vi "test drone.vi"() -> ()   [LabVIEW 2018]
uses:
  <vilib>/vision/Image Controls.llb/IMAQ Image.ctl
  <vilib>/Utility/error.llb/Error Cluster From Error Code.vi
  <vilib>/myRIO/Common/Instrument Driver Framework/myRIO v1.0/DIO/vis/myRIO v1.0 Write DIO.vi
  <vilib>/myRIO/Common/Instrument Driver Framework/myRIO v1.0/PWM/vis/myRIO v1.0 Write PWM.vi
  <vilib>/vision/driver/NI_Vision_Acquisition_Software.lvlib
  <vilib>/vision/NI_Vision_Development_Module.lvlib
  <vilib>/myRIO/Instrument Drivers/Onboard IO/PWM/PWM.lvlib
  <vilib>/myRIO/Instrument Drivers/Onboard IO/DIO/DIO.lvlib
panel:
  in  "Gimbal search":bool
  in  "Stop":bool
  out "Image 5":T1(plugin-control)
  out "Y":dbl[](array[numeric])
  out "X":dbl[](array[numeric])
  out "Antal isbjerg":i32
  out "logfile name":path
  in  "logfile base name":string="logfile"
  in  "Color Plane (Color Plane Extraction 1)":i32(ring)=1 items=["Red", "Green", "Blue", "Hue", "Saturation", "Luminance", "Value", "Intensity"]
  in  "Range (Threshold 1)":cluster{"Lower value":sgl, "Upper value":sgl}={"Lower value"=230.0, "Upper value"=255.0}
  in  "Structuring Element (Basic Morphology 1)":i32[][](array[numeric])=[[0, 1, 0], [1, 1, 1], [0, 1, 0]]
  in  "Number of Erosion (Advanced Morphology 1)":i32=12
  in  "Grounded?":bool
  in  "Pos. ROLL Boring":dbl
  in  "Pos. YAW Boring":dbl format="%#_13g"
  in  "Pos. ROLL No Search":dbl
  in  "Pos. YAW No Search":dbl format="%#_13g"
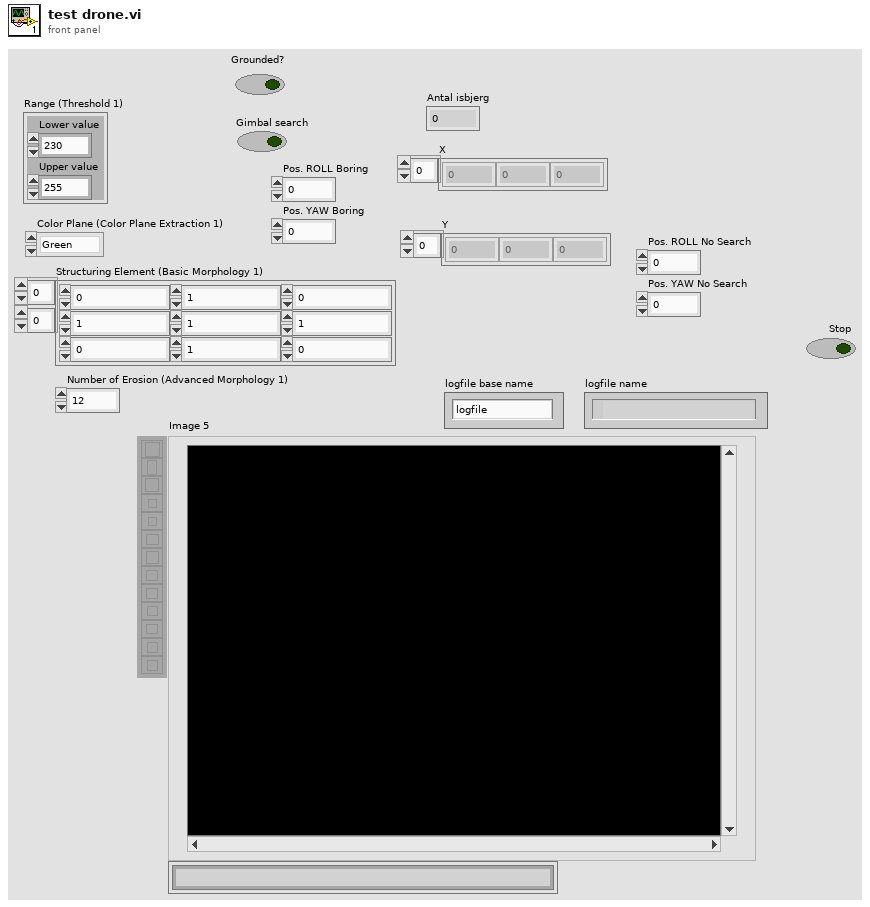
[diagram p1: front panel]
types:
  T1 = typedef "IMAQ Image.ctl" = refnum<image>
  T2 = typedef "DIO.lvlib/DIO Reference.ctl" = cluster{"myRIO Reference":T3, "DIO Channels List":T7}
  T3 = typedef "myRIO Generic Hardware Reference.ctl" = cluster{"myRIO Model":T4, "myRIO Hardware Reference":T5}
  T4 = typedef "Hardware Version Enum.ctl" = enum16{"Unknown", "myRIO-1900", "myRIO-1950", "roboRIO", "NI ELVIS RIO CM", "ELVIS III"}
  T5 = typedef "myRIO v1.0 Reference.ctl" = cluster{"Generic FPGA Reference":T6, "Allow multiple opens":bool}
  T6 = typedef "Generic FPGA Reference.ctl" = refnum<k20>
  T7 = typedef "DIO Channels List.ctl" = T8[]
  T8 = typedef "DIO Channels Enum.ctl" = enum16{"Not Connected", "C/DIO0", "C/DIO1", "C/DIO2", "C/DIO3", "C/DIO4", "C/DIO5", "C/DIO6", "C/DIO7", "A/DIO0", "A/DIO1", "A/DIO2", "A/DIO3", "A/DIO4", "A/DIO5", "A/DIO6", "A/DIO7", "A/DIO8", "A/DIO9", "A/DIO10", "A/DIO11", "A/DIO12", "A/DIO13", "A/DIO14", "A/DIO15", "A/DIO16", "A/DIO17", "A/DIO18", "A/DIO19", "B/DIO0", "B/DIO1", "B/DIO2", "B/DIO3", "B/DIO4", "B/DIO5", "B/DIO6", "B/DIO7", "B/DIO8", "B/DIO9", "B/DIO10", "B/DIO11", "B/DIO12", "B/DIO13", "B/DIO14", "B/DIO15", "B/DIO16", "B/DIO17", "B/DIO18", "B/DIO19", "LED0", "LED1", "LED2", "LED3", "Button0", "DIO/DIO0", "DIO/DIO1", "DIO/DIO2", "DIO/DIO3", "DIO/DIO4", "DIO/DIO5", "DIO/DIO6", "DIO/DIO7", "DIO/DIO8", "DIO/DIO9", "SPI/CS0", "SPI/CS1", "SPI/CS2", "SPI/CS3", "LED RADIO (Green)", "LED RADIO (Red)", "LED COMM (Green)", "LED COMM (Red)", "LED MODE (Green)", "LED MODE (Red)"}
  T9 = typedef "PWM.lvlib/PWM Reference.ctl" = cluster{"myRIO Reference":T3, "PWM Channels Enum":T10, "PWM Configuration":T11}
  T10 = typedef "PWM Channels Enum.ctl" = enum16{"Not Connected", "C/PWM0", "C/PWM1", "A/PWM0", "A/PWM1", "A/PWM2", "A/PWM3", "A/PWM4", "A/PWM5", "A/PWM6", "A/PWM7", "A/PWM8", "A/PWM9", "A/PWM10", "A/PWM11", "A/PWM12", "A/PWM13", "A/PWM14", "A/PWM15", "A/PWM16", "A/PWM17", "A/PWM18", "A/PWM19", "B/PWM0", "B/PWM1", "B/PWM2", "B/PWM3", "B/PWM4", "B/PWM5", "B/PWM6", "B/PWM7", "B/PWM8", "B/PWM9", "B/PWM10", "B/PWM11", "B/PWM12", "B/PWM13", "B/PWM14", "B/PWM15", "B/PWM16", "B/PWM17", "B/PWM18", "B/PWM19", "PWM/PWM0", "PWM/PWM1", "PWM/PWM2", "PWM/PWM3", "PWM/PWM4", "PWM/PWM5", "PWM/PWM6", "PWM/PWM7", "PWM/PWM8", "PWM/PWM9"}
  T11 = typedef "PWM.lvlib/PWM Configuration.ctl" = cluster{"Frequency":dbl, "Duty Cycle":dbl}
  T12 = typedef "Accelerometer.lvlib/Accelerometer Reference.ctl" = cluster{"myRIO Reference":T3, "Accelerometer Channels List":T13, "LSB Weight":dbl}
  T13 = typedef "Accelerometer Channels List.ctl" = T14[]
  T14 = typedef "Accelerometer Channels Enum.ctl" = enum16{"Not Connected", "X-Axis", "Y-Axis", "Z-Axis"}
  T15 = typedef "AI.lvlib/AI Reference.ctl" = cluster{"myRIO Reference":T3, "AI Channels List":T16, "AI Scaling Constants List":T18}
  T16 = typedef "AI Channels List.ctl" = T17[]
  T17 = typedef "AI Channels Enum.ctl" = enum16{"Not Connected", "AudioIn/Left", "AudioIn/Right", "C/AI0", "C/AI1", "A/AI0", "A/AI1", "A/AI2", "A/AI3", "A/AI4", "A/AI5", "A/AI6", "A/AI7", "B/AI0", "B/AI1", "B/AI2", "B/AI3", "B/AI4", "B/AI5", "B/AI6", "B/AI7", "AI/AI0", "AI/AI1", "AI/AI2", "AI/AI3", "A/AI0 (DIFF)", "A/AI1 (DIFF)", "A/AI2 (DIFF)", "A/AI3 (DIFF)", "B/AI0 (DIFF)", "B/AI1 (DIFF)", "B/AI2 (DIFF)", "B/AI3 (DIFF)"}
  T18 = typedef "Analog Scaling Constants List.ctl" = T19[]
  T19 = typedef "Analog Scaling Constants.ctl" = cluster{"LSB Weight (Volts)":dbl, "Offset (Volts)":dbl, "Signed?":bool}
  T20 = typedef "SPI.lvlib/SPI Reference.ctl" = cluster{"myRIO Reference":T3, "SPI Channels Enum":T21, "SPI Configuration":T22}
  T21 = typedef "SPI Channels Enum.ctl" = enum16{"Not Connected", "A/SPI", "B/SPI", "SPI/SPI"}
  T22 = typedef "SPI.lvlib/SPI Configuration.ctl" = cluster{"Frequency [Hz]":dbl, "Clock Phase":T23, "Clock Polarity":T24, "Data Direction":T25, "Frame Length":T26}
  T23 = typedef "SPI Clock Phase.ctl" = enum8{"Leading", "Trailing"}
  T24 = typedef "SPI Clock Polarity.ctl" = enum8{"Low", "High"}
  T25 = typedef "SPI Data Direction.ctl" = enum8{"Most significant bit first", "Least significant bit first"}
  T26 = typedef "SPI Frame Length.ctl" = u8
  T27 = cluster{"B/DIO0 - Stepper Direction":T2, "B/DIO1 - Stepper1 Enable":T2, "B/DIO2 - Stepper2 Enable":T2, "B/DIO3 - Stepper3 Enable":T2, "B/DIO4 - Endstop Stepper1 Top":T2, "B/DIO11 - Endstop Stepper1 Bund":T2, "B/DIO12 - Endstop Stepper2 Top":T2, "B/DIO13 - Endstop Stepper2 Bund":T2, "B/DIO14 - Endstop Stepper3 Top":T2, "B/DIO15 - Endstop Stepper3 Bund":T2, "A/DIO0 - Cooler":T2, "A/DIO1 - Beacon drop (dio1)":T2, "A/DIO2 - Beacon drop (dio0)":T2, "A/DIO3 - QuickRelease (dio1)":T2, "A/DIO4 - QuickRelease (dio0)":T2, "A/DIO11 - LiDAR SPI CS":T2, "B/PWM0 - Stepper":T9, "B/PWM1 - Drill":T9, "A/PWM0 - Servo_Roll":T9, "A/PWM1 - Servo_Yaw":T9, "Acc. X-axis":T12, "Acc. Y-axis":T12, "B/AI0 - Drone Grounded F3":T15, "B/AI1 - Drone Drill Gear F4":T15, "B/AI2 - Beacon Drop F5":T15, "B/AI3 - Drone Drill Boost F6":T15, "A/AI0 - Drone Stepper F8":T15, "A/AI1 - Beacon Wiper":T15, "A/AI2 - QuickRelease Wiper":T15, "A/AI3 - Drill Current":T15, "A/SPI - LiDAR":T20, "B/UART - XBee":refnum<visa-resource-name>, "A/UART - A3 GPS":refnum<visa-resource-name>, "RIO Flashing LEDs":T2}
  T28 = enum32{"AutoM", "Close", "Dilate", "Erode", "Gradient", "Gradient out", "Gradient in", "Hit miss", "Open", "PClose", "POpen", "Thick", "Thin"}
  T29 = typedef "Image Type" = u32
  T30 = typedef "IMAQdx.ctl" = refnum<k21>
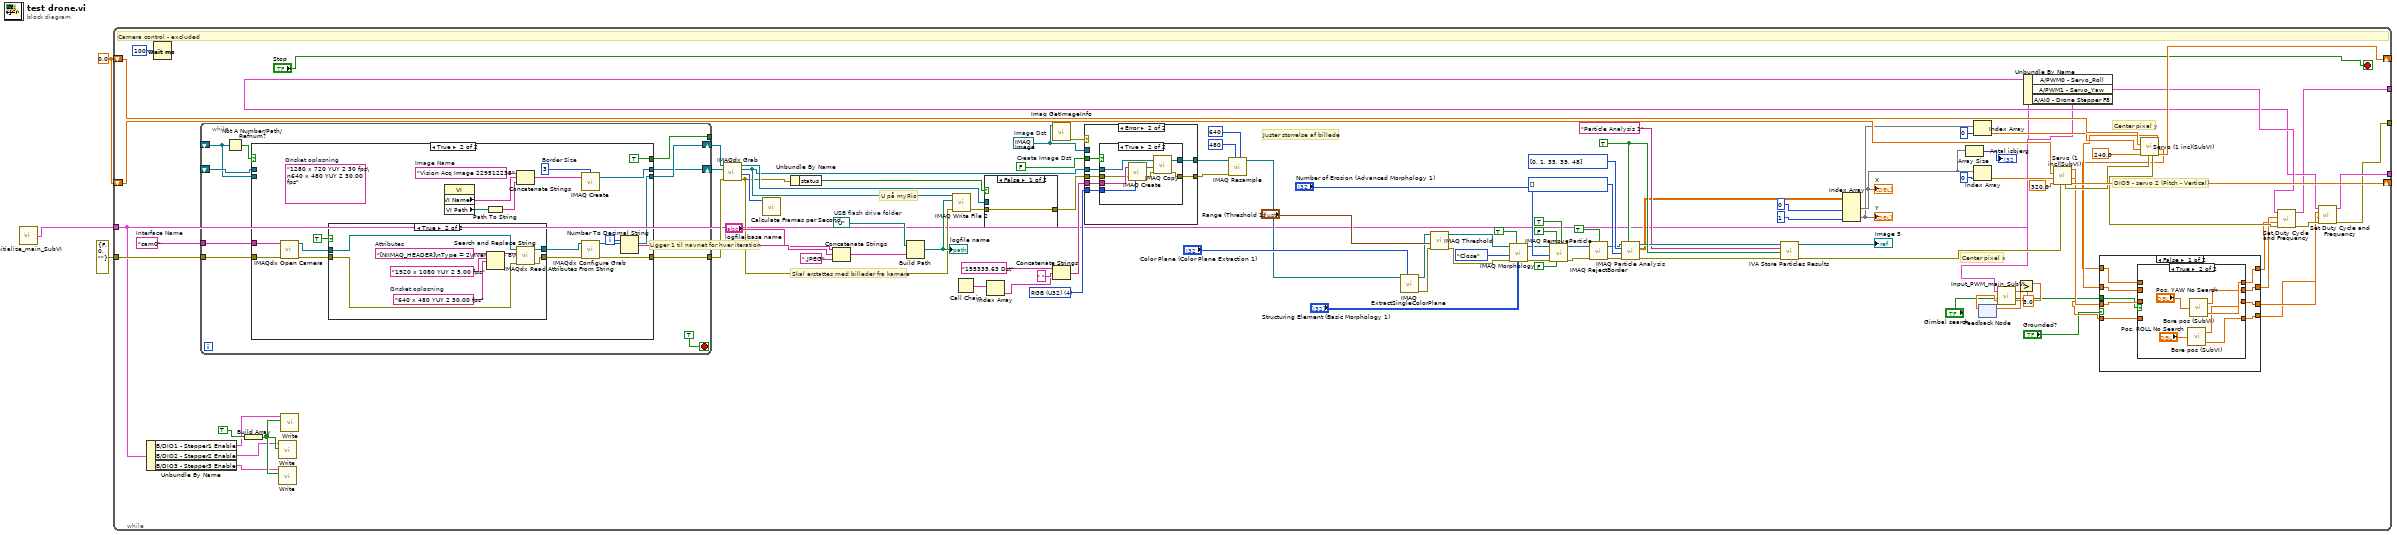
[diagram p0: block diagram]
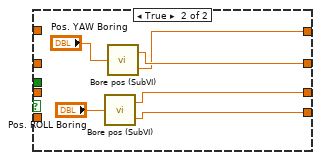
[diagram p3: hidden frame]
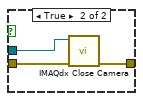
[diagram p4: hidden frame]
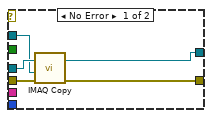
[diagram p7: hidden frame]
diagram:
  w1 = 0.0 ("Position 2")
  n1 = call "Initialize_main_SubVI.vi"() -> ("output cluster"=w3:T27)
  n2 = while {
    shift-right: [w78] -> _
    shift-left: w1 -> [w81]
    shift-right: [w93] -> _
    shift-left: w1 -> [w94]
    tunnel: errorcluster {"status"=FALSE, "code"=0, "source"=""} ("error out") -> [w95]
    tunnel: w3 -> [w10]
    tunnel: [w30] -> _
    tunnel: [w34] -> _
    tunnel: [w33] -> _
    i -> [w68]
    stop <- "Stop" stop-if-true
    w46 = i32[] [] items=["Center of Mass X", "Center of Mass Y", "First Pixel X", "First Pixel Y", "Bounding Rect Left", "Bounding Rect Top", "Bounding Rect Right", "Bounding Rect Bottom", "Max Feret Diameter Start X", "Max Feret Diameter Start Y", "Max Feret Diameter End X", "Max Feret Diameter End Y", "Max Horiz. Segment Length Left", "Max Horiz. Segment Length Right", "Max Horiz. Segment Length Row", "-", "Bounding Rect Width", "Bounding Rect Height", "Bounding Rect Diagonal", "Perimeter", "Convex Hull Perimeter", "Holes' Perimeter", "Max Feret Diameter", "Equivalent Ellipse Major Axis", "Equivalent Ellipse Minor Axis", "Equivalent Ellipse Minor Axis (Feret)", "Equivalent Rect Long Side", "Equivalent Rect Short Side", "Equivalent Rect Diagonal", "Equivalent Rect Short Side (Feret)", "Average Horiz. Segment Length", "Average Vert. Segment Length", "Hydraulic Radius", "Waddel Disk Diameter", "-", "Area", "Holes' Area", "Particle & Holes' Area", "Convex Hull Area", "Image Area", "-", "Number of Holes", "Number of Horiz. Segments", "Number of Vert. Segments", "-", "Orientation", "Max Feret Diameter Orientation", "-", "% Area/Image Area", "% Area/(Particle & Holes' Area)", "Ratio of Equivalent Ellipse Axes", "Ratio of Equivalent Rect Sides", "-", "Elongation Factor", "Compactness Factor", "Heywood Circularity Factor", "Type Factor", "-", "Sum X", "Sum Y", "Sum XX", "Sum XY", "Sum YY", "Sum XXX", "Sum XXY", "Sum XYY", "Sum YYY", "-", "Moment of Inertia XX", "Moment of Inertia XY", "Moment of Inertia YY", "Moment of Inertia XXX", "Moment of Inertia XXY", "Moment of Inertia XYY", "Moment of Inertia YYY", "Norm. Moment of Inertia XX", "Norm. Moment of Inertia XY", "Norm. Moment of Inertia YY", "Norm. Moment of Inertia XXX", "Norm. Moment of Inertia XXY", "Norm. Moment of Inertia XYY", "Norm. Moment of Inertia YYY", "Hu Moment 1", "Hu Moment 2", "Hu Moment 3", "Hu Moment 4", "Hu Moment 5", "Hu Moment 6", "Hu Moment 7"] ("Real-World Measurements")
    w47 = i32[] [0, 1, 35, 39, 48] items=["Center of Mass X", "Center of Mass Y", "First Pixel X", "First Pixel Y", "Bounding Rect Left", "Bounding Rect Top", "Bounding Rect Right", "Bounding Rect Bottom", "Max Feret Diameter Start X", "Max Feret Diameter Start Y", "Max Feret Diameter End X", "Max Feret Diameter End Y", "Max Horiz. Segment Length Left", "Max Horiz. Segment Length Right", "Max Horiz. Segment Length Row", "-", "Bounding Rect Width", "Bounding Rect Height", "Bounding Rect Diagonal", "Perimeter", "Convex Hull Perimeter", "Holes' Perimeter", "Max Feret Diameter", "Equivalent Ellipse Major Axis", "Equivalent Ellipse Minor Axis", "Equivalent Ellipse Minor Axis (Feret)", "Equivalent Rect Long Side", "Equivalent Rect Short Side", "Equivalent Rect Diagonal", "Equivalent Rect Short Side (Feret)", "Average Horiz. Segment Length", "Average Vert. Segment Length", "Hydraulic Radius", "Waddel Disk Diameter", "-", "Area", "Holes' Area", "Particle & Holes' Area", "Convex Hull Area", "Image Area", "-", "Number of Holes", "Number of Horiz. Segments", "Number of Vert. Segments", "-", "Orientation", "Max Feret Diameter Orientation", "-", "% Area/Image Area", "% Area/(Particle & Holes' Area)", "Ratio of Equivalent Ellipse Axes", "Ratio of Equivalent Rect Sides", "-", "Elongation Factor", "Compactness Factor", "Heywood Circularity Factor", "Type Factor", "-", "Sum X", "Sum Y", "Sum XX", "Sum XY", "Sum YY", "Sum XXX", "Sum XXY", "Sum XYY", "Sum YYY", "-", "Moment of Inertia XX", "Moment of Inertia XY", "Moment of Inertia YY", "Moment of Inertia XXX", "Moment of Inertia XXY", "Moment of Inertia XYY", "Moment of Inertia YYY", "Norm. Moment of Inertia XX", "Norm. Moment of Inertia XY", "Norm. Moment of Inertia YY", "Norm. Moment of Inertia XXX", "Norm. Moment of Inertia XXY", "Norm. Moment of Inertia XYY", "Norm. Moment of Inertia YYY", "Hu Moment 1", "Hu Moment 2", "Hu Moment 3", "Hu Moment 4", "Hu Moment 5", "Hu Moment 6", "Hu Moment 7"] ("Pixel Measurements")
    w44 = TRUE ("Connectivity 4/8 (8)")
    w67 = path "U:/"  # USB flash drive folder
    w101 = "cam0"  # Interface Name
    w111 = T1 refnum  # Image Dst
    w103 = T29 4 items=["Grayscale (U8)", "Grayscale (I16)", "Grayscale (SGL)", "Complex (CSG)", "RGB (U32)", "HSL (U32)", "RGB (U64)", "Grayscale (U16)"] ("Image Dst Type")
    w109 = FALSE  # Create Image Dst
    # "Juster størrelse af billede"
    # "U på myRio"
    # "Ligger 1 til navnet for hver iteration"
    # "Skal erstattes med billeder fra kamera"
    # "Center pixel y"
    # "Center pixel x"
    # "DIO9 - servo 2 (Pitch - Vertical)"
    # "Camera control - excluded"
    n3 = Unbundle By Name(w10) -> ("B/DIO1 - Stepper1 Enable"=w7:T2, "B/DIO2 - Stepper2 Enable"=w6:T2, "B/DIO3 - Stepper3 Enable"=w5:T2)
    n4 = Wait (ms)(milliseconds to wait=u32 100) -> ()  [unwired: 1 out]
    n5 = while "While Loop_template0" {
      shift-right: [w150] -> w96
      shift-left: _ -> [w143]
      tunnel: [w149] -> w102
      tunnel: w95 -> [w148]
      shift-right: [w146] -> w97
      shift-left: _ -> [w145]
      tunnel: w101 -> [w144]
      tunnel: [w141] -> _
      stop <- TRUE ("_template0") stop-if-true
      n6 = Not A Number/Path/Refnum?(number/path/refnum=w143) -> (NaN/Path/Refnum?=w142:bool)
      n7 = case "Case Structure_template0" shown="True" w142 {
        tunnel: [w153 w169] -> w150
        tunnel: w143 -> [w153 _]
        tunnel: [w152 w168] -> w149
        tunnel: w148 -> [w152 w170]
        tunnel: [w151 w167] -> w146
        tunnel: w145 -> [w151 _]
        tunnel: w144 -> [_ w158]
        tunnel: [_ TRUE] -> w141
        frame False {
        }
        frame True {
          (unwired) "1280 x 720 YUY 2 30 fps\n640 x 480 YUY 2 30.00 fps"  # Ønsket opløsning
          w155 = 3  # Border Size
          w162 = "Vision Acq Image 229512235"  # Image Name
          n8 = call <vilib>:"IMAQdx Open Camera.vi"("error in"=w170, "Session In"=w158) -> ("error out"=w160:errorcluster, "Session Out"=w161:T30)  [unwired: 1 in, 7 out]
          n9 = case shown="True" TRUE ("Init Attributes") {
            tunnel: w161 -> [w172 w180]
            tunnel: w160 -> [w171 w179]
            tunnel: [w172 w178] -> w154
            tunnel: [w171 w177] -> w159
            frame False {
            }
            frame True {
              w173 = "640 x 480 YUY 2 30.00 fps"  # Ønsket opløsning
              w176 = "[NIIMAQ_HEADER]\nType = 2\nVersion = 8\n\n[CAMERA_DATA]\nAcquisitionAttributes::Bayer::Algorithm = \"Bilinear\"\nAcquisitionAttributes::Bayer::GainB = \"1\"\nAcquisitionAttributes::Bayer::GainG = \"1\"\nAcquisitionAttributes::Bayer::GainR = \"1\"\nAcquisitionAttributes::Bayer::Pattern = \"Use hardware value\"\nAcquisitionAttributes::BitsPerPixel = \"Use hardware value\"\nAcquisitionAttributes::HardwareMaximumQueuedBufferCount = \"1000\"\nAcquisitionAttributes::HardwareRequeueBufferListThreshold = \"50\"\nAcquisitionAttributes::IgnoreFirstFrame = \"false\"\nAcquisitionAttributes::ImageDecoderCopyMode = \"Auto\"\nAcquisitionAttributes::OutputImageType = \"Auto\"\nAcquisitionAttributes::OverwriteMode = \"Get Newest\"\nAcquisitionAttributes::PixelSignedness = \"Use hardware value\"\nAcquisitionAttributes::ReceiveTimestampMode = \"None\"\nAcquisitionAttributes::ShiftPixelBits = \"false\"\nAcquisitionAttributes::SwapPixelBytes = \"false\"\nAcquisitionAttributes::Timeout = \"5000\"\nAcquisitionAttributes::VideoMode = \"1920 x 1080 YUY 2 5.00 fps\"\nCameraAttributes::BacklightCompensation::Mode = \"Manual\"\nCameraAttributes::BacklightCompensation::Value = \"0\"\nCameraAttributes::Brightness::Mode = \"Manual\"\nCameraAttributes::Brightness::Value = \"168\"\nCameraAttributes::Contrast::Mode = \"Manual\"\nCameraAttributes::Contrast::Value = \"5\"\nCameraAttributes::Exposure::Mode = \"AutoAperaturePriority\"\nCameraAttributes::Focus::Mode = \"Auto\"\nCameraAttributes::Pan::Mode = \"Manual\"\nCameraAttributes::Pan::Value = \"0\"\nCameraAttributes::PowerLineFrequency::Mode = \"60Hz\"\nCameraAttributes::Saturation::Mode = \"Manual\"\nCameraAttributes::Saturation::Value = \"103\"\nCameraAttributes::Sharpness::Mode = \"Manual\"\nCameraAttributes::Sharpness::Value = \"25\"\nCameraAttributes::Tilt::Mode = \"Manual\"\nCameraAttributes::Tilt::Value = \"0\"\nCameraAttributes::WhiteBalance::Mode = \"Auto\"\nCameraAttributes::Zoom::Mode = \"Manual\"\nCameraAttributes::Zoom::Value = \"0\"\n"  # Attributes
              n10 = Search and Replace String(input string=w176, search string="1920 x 1080 YUY 2 5.00 fps", replace string=w173) -> (result string=w174:string)  [unwired: 5 in, 3 out]
              n11 = call <vilib>:"IMAQdx Read Attributes From String.vi"("error in"=w179, "Attributes String In"=w174, "Session In"=w180) -> ("error out"=w177:errorcluster, "Session Out"=w178:T30)  [unwired: 7 out]
            }
          }
          n12 = property class="VI"() -> ("VI Name"=w165:string, "VI Path"=w166:path)  [unwired: 2 in, 2 out]
          n13 = Path To String(path=w166) -> (string=w164:string)
          n14 = Concatenate Strings(w162, w165, w164) -> (w163:string)
          n15 = call "IMAQ Create"("Border Size"=w155, "Image Name"=w163) -> ("New Image"=w167:T1)  [unwired: 2 in, 2 out]
          n16 = call <vilib>:"IMAQdx Configure Grab.vi"("error in"=w159, "Session In"=w154) -> ("error out"=w168:errorcluster, "Session Out"=w169:T30)  [unwired: 8 out]
        }
      }
    }
    n17 = Build Array(TRUE) -> (w8:bool[])
    n18 = call <vilib>:"Write.vi"("Values"=w8, "DIO Ref In"=w6) -> ()  [unwired: 7 in, 2 out]
    n19 = call <vilib>:"Write.vi"("Values"=w8, "DIO Ref In"=w5) -> ()  [unwired: 7 in, 2 out]
    n20 = call <vilib>:"Write.vi"("Values"=w8, "DIO Ref In"=w7) -> ()  [unwired: 7 in, 2 out]
    n21 = Number To Decimal String(number=w68) -> (decimal integer string=w73:string)  [unwired: 1 in]
    n22 = call <vilib>:"IMAQdx Grab.vi"("error in"=w102, "Image In"=w97, "Session In"=w96) -> ("error out"=w70:errorcluster, "Buffer Number Out"=w100:u32, "Image Out"=w71:T1, "Session Out"=w99:T30)  [unwired: 1 in, 4 out]
    n23 = call <vilib>:"Calculate Frames per Second.vi"("Buffer Number"=w100) -> ()  [unwired: 2 in, 9 out]
    n24 = Unbundle By Name(w70) -> ("status"=w90:bool)
    n25 = Concatenate Strings "Concatenate Strings"("logfile base name", w73, ".JPEG" ("string")) -> (w75:string)
    n26 = Build Path(base path=w67, name or relative path=w75) -> (appended path=w76:path)
    "logfile name" <- w76
    n27 = call-poly "IMAQ Write File 2"("error in (no error)"=w70, "File Path"=w76, "Image"=w71) -> ("error out"=w69:errorcluster)  [unwired: 7 in, 1 out]
    n28 = Call Chain() -> (call chain=w108:string[])
    n29 = case "Case Structure_template1" shown="False" w90 {
      tunnel: [w137 w139] -> w98
      tunnel: w69 -> [w137 w140]
      tunnel: w99 -> [_ w138]
      frame False {
      }
      frame True {
        n30 = call <vilib>:"IMAQdx Close Camera.vi"("error in"=w140, "Session In"=w138) -> ("error out"=w139:errorcluster)  [unwired: 9 out]
      }
    }
    n31 = Index Array(array=w108) -> (element=w106:string)  [unwired: 1 in]
    n32 = call "Imaq GetImageInfo"("Image"=w111) -> ("error out"=w110:errorcluster)  [unwired: 1 in, 9 out]
    n33 = Concatenate Strings("155335,63 Dst" ("Image Dst Name"), " ", w106) -> (w104:string)
    n34 = case shown="Error" w110 {
      tunnel: [w185 w189] -> w38
      tunnel: [w184 w188] -> w37
      tunnel: w71 -> [w183 w190]
      tunnel: w98 -> [w182 w186]
      tunnel: w111 -> [w181 _]
      tunnel: w104 -> [_ w192]
      tunnel: w103 -> [_ w191]
      tunnel: w109 -> [_ w187]
      frame No Error {
        n35 = call "IMAQ Copy"("error in (no error)"=w182, "Image Dst"=w181, "Image Src"=w183) -> ("error out"=w184:errorcluster, "Image Dst Out"=w185:T1)  [unwired: 3 out]
      }
      frame Error {
        n36 = case shown="True" w187 {
          tunnel: w192 -> [_ w202]
          tunnel: w191 -> [_ w201]
          tunnel: w190 -> [w194 w199]
          tunnel: [w194 w198] -> w189
          tunnel: [w193 w197] -> w188
          tunnel: w186 -> [w193 w195]
          frame False {
          }
          frame True {
            n37 = call "IMAQ Create"("Image Name"=w202, "Image Type"=w201, "error in (no error)"=w195) -> ("New Image"=w200:T1, "error out"=w196:errorcluster)  [unwired: 1 in, 1 out]
            n38 = call "IMAQ Copy"("error in (no error)"=w196, "Image Dst"=w200, "Image Src"=w199) -> ("error out"=w197:errorcluster, "Image Dst Out"=w198:T1)  [unwired: 3 out]
          }
        }
      }
    }
    n39 = call "IMAQ Resample"("X Resolution"=u16 640 ("Width"), "Y Resolution"=u16 480 ("Height"), "error in (no error)"=w37, "Image Src"=w38) -> ("Image Dst Out"=w14:T1)  [unwired: 6 in, 1 out]
    n40 = call "IMAQ ExtractSingleColorPlane"("Color Plane"="Color Plane (Color Plane Extraction 1)", "Image Src"=w14) -> ("error out"=w65:errorcluster, "Image Dst Out"=w63:T1)  [unwired: 2 in, 6 out]
    n41 = call "IMAQ Threshold"("error in (no error)"=w65, "Range"="Range (Threshold 1)", "Image Src"=w63) -> ("error out"=w62:errorcluster, "Image Dst Out"=w58:T1)  [unwired: 3 in, 4 out]
    n42 = call "IMAQ Morphology"("Structuring Element"="Structuring Element (Basic Morphology 1)", "Square/Hexa (Square)"=TRUE, "error in (no error)"=w62, "Operation"=T28."Close", "Image Src"=w58) -> ("error out"=w57:errorcluster, "Image Dst Out"=w52:T1)  [unwired: 2 in, 3 out]
    n43 = call "IMAQ RemoveParticle"("Connectivity 4/8 (8)"=TRUE, "Low Pass/High Pass (Low)"=FALSE, "Square/Hexa (Square)"=FALSE, "error in (no error)"=w57, "Number of Erosion"="Number of Erosion (Advanced Morphology 1)", "Image Src"=w52) -> ("error out"=w51:errorcluster, "Image Dst Out"=w49:T1)  [unwired: 1 in, 3 out]
    n44 = call "IMAQ RejectBorder"("error in (no error)"=w51, "Image Src"=w49, "Connectivity 4/8 (8)"=TRUE) -> ("error out"=w48:errorcluster, "Image Dst Out"=w45:T1)  [unwired: 1 in, 2 out]
    n45 = call "IMAQ Particle Analysis"("Connectivity 4/8 (8)"=w44, "error in (no error)"=w48, "Real-World Measurements"=w46, "Pixel Measurements"=w47, "Image"=w45) -> ("error out"=w41:errorcluster, "Particle Measurements (Pixels)"=w39:dbl[][], "Image Out (duplicate)"=w43:T1)  [unwired: 4 out]
    n46 = call <vilib>:"IVA Store Particles Results.vi"("error in (no error)"=w41, "Connectivity 4/8 (8)"=w44, "Step Name"="Particle Analysis 1", "Image in"=w43) -> ("error out"=w40:errorcluster, "Image dup"=→"Image 5":T1)  [unwired: 6 out]
    n47 = Index Array(array=w39, index (col) #1=0 ("index (col)"), index (col) #2=1 ("index (col)")) -> (element #1=w85:dbl[], element #2=w82:dbl[])  [unwired: 2 in]
    "Y" <- w82
    "X" <- w85
    n48 = Array Size(array=w85) -> (size(s)=→"Antal isbjerg":i32)
    n49 = Index Array(array=w82, index=0) -> (element=w77:dbl)
    n50 = Index Array(array=w85, index=0) -> (element=w84:dbl)
    n51 = feedback #1() -> (w19:dbl[])  [unwired: 1 in]
    n52 = Unbundle By Name(w10) -> ("A/PWM0 - Servo_Roll"=w35:T9, "A/PWM1 - Servo_Yaw"=w36:T9, "A/AI0 - Drone Stepper F8"=w21:T15)
    n53 = call "Input_PWM_main_SubVI.vi"("Shift in"=w19, "AI Ref In"=w21) -> ("Value out"=w18:dbl, "Shift out"=w20:dbl[])
    n54 = feedback-in #1(w20) -> ()
    n55 = Greater?(x=w18, y=3.0) -> ()  [unwired: 1 out]
    n56 = call "Servo (1 inc)(SubVI).vi"("error constant 2"=w40, "Center pixel"=320.0 ("Center pixel 2"), "Pixel value"=w84, "Position."=w94) -> ("Position 2"=w93:dbl, "freq [Hz]"=w22:dbl, "Duty"=w26:dbl, "error constant"=w79:errorcluster)  [unwired: 3 in, 1 out]
    n57 = call "Servo (1 inc)(SubVI).vi"("error constant 2"=w79, "Center pixel"=240.0, "Pixel value"=w77, "Position."=w81) -> ("Position 2"=w78:dbl, "freq [Hz]"=w24:dbl, "Duty"=w28:dbl, "error constant"=w32:errorcluster)  [unwired: 3 in, 1 out]
    n58 = case shown="False" "Grounded?" {
      tunnel: [w118 w135] -> w29
      tunnel: w28 -> [w117 _]
      tunnel: [w116 w136] -> w27
      tunnel: w26 -> [w115 _]
      tunnel: [w120 w134] -> w25
      tunnel: w24 -> [w119 _]
      tunnel: [w114 w133] -> w23
      tunnel: w22 -> [w113 _]
      tunnel: "Gimbal search" -> [w112 _]
      frame False {
        n59 = case shown="True" w112 {
          tunnel: [w124 w127] -> w120
          tunnel: w119 -> [w124 _]
          tunnel: [w123 w126] -> w118
          tunnel: w117 -> [w123 _]
          tunnel: [w122 w125] -> w116
          tunnel: w115 -> [w122 _]
          tunnel: [w121 w128] -> w114
          tunnel: w113 -> [w121 _]
          frame False {
          }
          frame True {
            n60 = call "Bore pos (SubVI).vi"("Position."="Pos. ROLL No Search") -> ("Duty"=w125:dbl, "freq [Hz]"=w128:dbl)
            n61 = call "Bore pos (SubVI).vi"("Position."="Pos. YAW No Search") -> ("Duty"=w126:dbl, "freq [Hz]"=w127:dbl)
          }
        }
      }
      frame True {
        n62 = call "Bore pos (SubVI).vi"("Position."="Pos. ROLL Boring") -> ("Duty"=w136:dbl, "freq [Hz]"=w133:dbl)
        n63 = call "Bore pos (SubVI).vi"("Position."="Pos. YAW Boring") -> ("Duty"=w135:dbl, "freq [Hz]"=w134:dbl)
      }
    }
    n64 = call <vilib>:"Set Duty Cycle and Frequency.vi"("error in (no error)"=w32, "Frequency [Hz]"=w25, "Duty Cycle"=w29, "PWM Ref In"=w36) -> ("error out"=w31:errorcluster, "PWM Ref Out"=w34:T9)  [unwired: 5 in]
    n65 = call <vilib>:"Set Duty Cycle and Frequency.vi"("error in (no error)"=w31, "Frequency [Hz]"=w23, "Duty Cycle"=w27, "PWM Ref In"=w35) -> ("error out"=w30:errorcluster, "PWM Ref Out"=w33:T9)  [unwired: 5 in]
  }
